vi "Polar to Cartesian.vi"(4 "Polar\nCoordinates":cluster{"r":dbl, "theta":dbl}) -> (1 "Cartesian\nCoordinates":cluster{"x":dbl, "y":dbl})   [LabVIEW 2013]
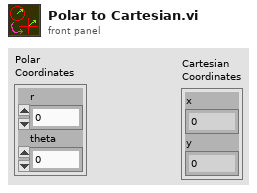
[diagram p1: front panel]
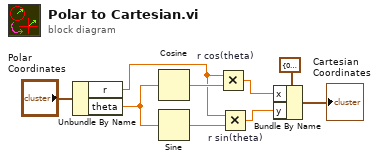
[diagram p0: block diagram]
diagram:
  n1 = Unbundle By Name("Polar\nCoordinates") -> ("r"=w1:dbl, "theta"=w2:dbl)
  n2 = Cosine(x=w2) -> (cos(x)=w9:dbl)
  n3 = Sine(x=w2) -> (sin(x)=w8:dbl)
  n4 = Multiply "r cos(theta)"(x=w1, y=w9) -> (x*y=w5:dbl)
  n5 = Multiply "r sin(theta)"(x=w1, y=w8) -> (x*y=w4:dbl)
  n6 = Bundle By Name(cluster=cluster{"x":dbl, "y":dbl} {"x"=0.0, "y"=0.0} ("input cluster"), "x"=w5, "y"=w4) -> (→"Cartesian\nCoordinates":cluster{"x":dbl, "y":dbl})
